vi "git_add_all.vi"(8 "Error In":errorcluster, 10 "Working Directory In":path=path "", 11 "add_all_button":bool) -> (0 "Error Out":errorcluster, 1 "standard output":string, 2 "Working Directory Out":path, 3 "add_all_indicator":bool)   [LabVIEW 2026]
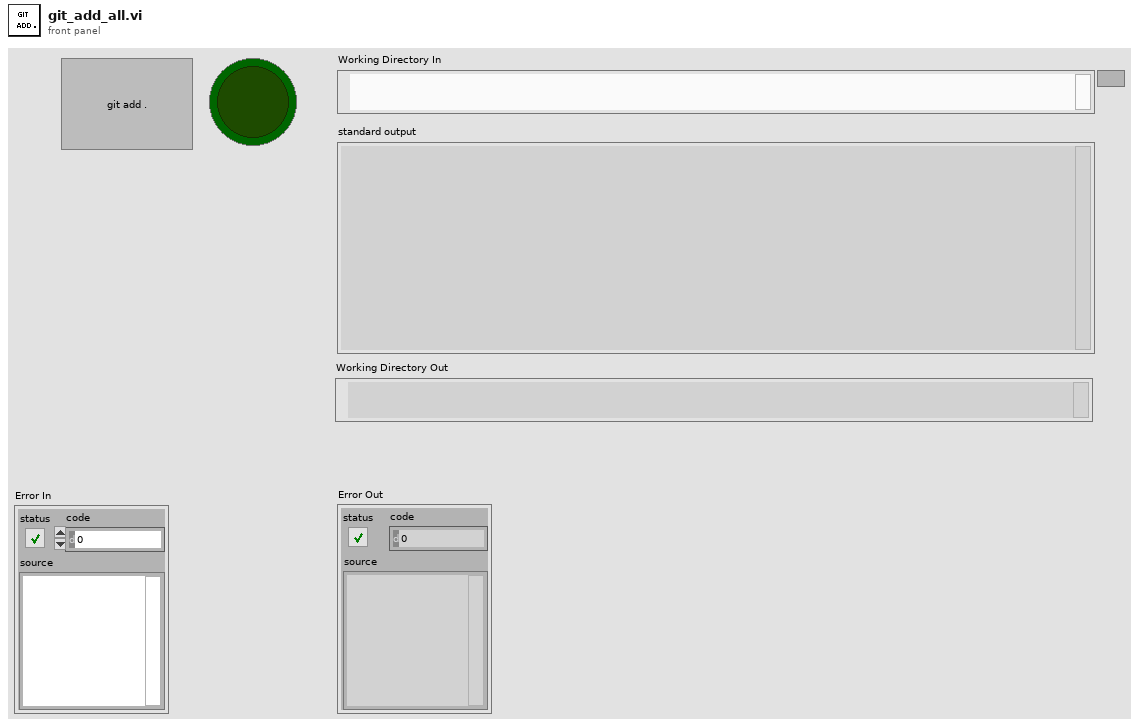
[diagram p1: front panel]
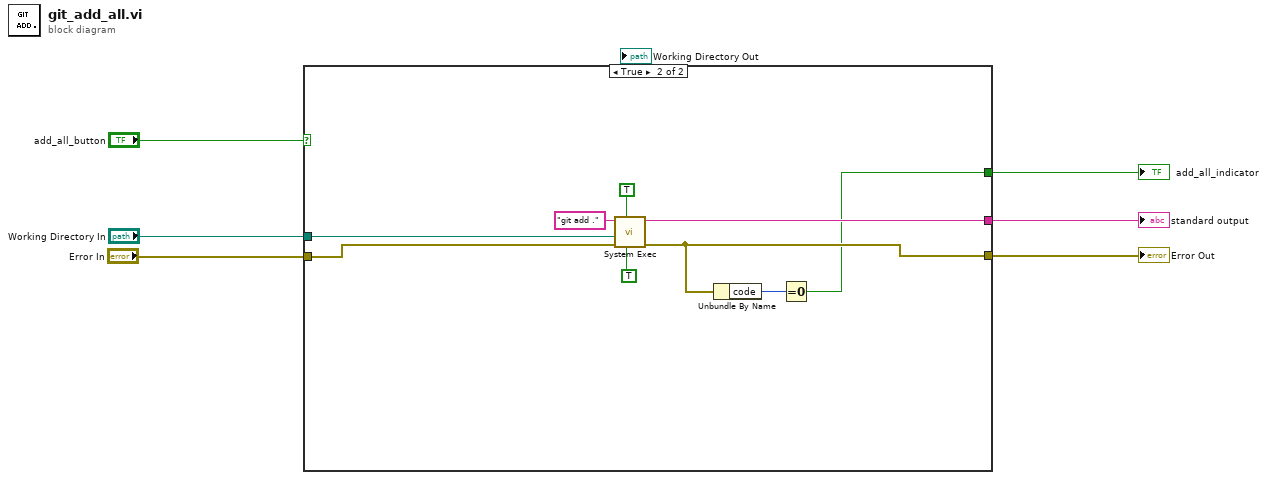
[diagram p0: block diagram]
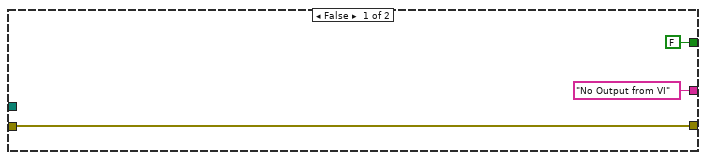
[diagram p2: hidden frame]
diagram:
  n1 = case shown="True" "add_all_button" {
    tunnel: "Working Directory In" -> [_ w18]
    tunnel: "Error In" -> [w7 w16]
    tunnel: [w7 w12] -> w4
    tunnel: ["No Output from VI" ("standard output") w14] -> w3
    tunnel: [FALSE w10] -> w2
    frame False {
    }
    frame True {
      n2 = call <vilib>:"System Exec.vi"("run minimized? (F)"=TRUE, "wait until completion? (T)"=TRUE, "error in (no error)"=w16, "working directory"=w18, "command line"="git add .") -> ("error out"=w12:errorcluster, "standard output"=w14:string)  [unwired: 3 in, 2 out]
      n3 = Unbundle By Name(w12) -> ("code"=w11:i32)
      n4 = Equal To 0?(x=w11) -> (x = 0?=w10:bool)
    }
  }
  "Error Out" <- w4
  "standard output" <- w3
  "add_all_indicator" <- w2
